vi "PPMS_Measure_v2.vi"(6 "error in (no error)":errorcluster, 7 "Index":i8) -> (0 "error out":errorcluster, 2 "resulting string 1":string="Measure Lockin Channe1, Channel2,  Averages 0 every 0 seconds", 3 "Cancelled?":bool=TRUE)   [LabVIEW 2017]
doc: "Use this template to create a dialog box. This template polls the state of the buttons on the front panel and does not use events. Use the Dialog Using Events template (not available in Base package) to create a dialog box with event handling."
panel:
  in  "Meas Time (s)":dbl=10.0
  in  "Stability timeout (s)":dbl=10.0
  out "MODE":i32(ring) items=["SET&MEAS", "SCAN", ""]
  in  "Measure Rate (s)":dbl=1.0 format="%.3f"
  in  "Averages":u16=10
  in  "Cancel":bool
  in  "OK":bool
  # "Noviembre 2020 V1.2  a-sslcdms"
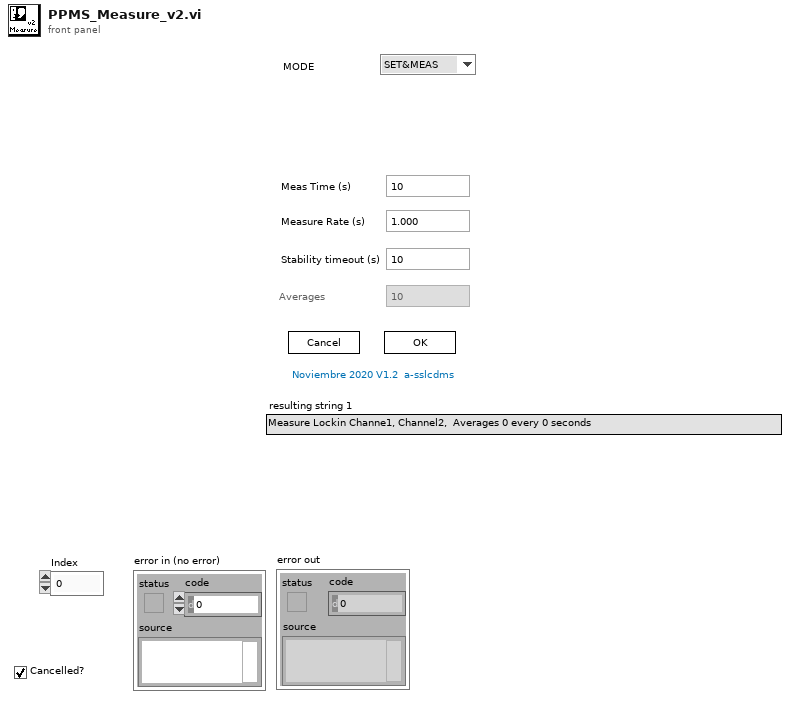
[diagram p1: front panel]
types:
  T1 = enum8{"Enabled", "Disabled", "Disabled and Grayed Out"}
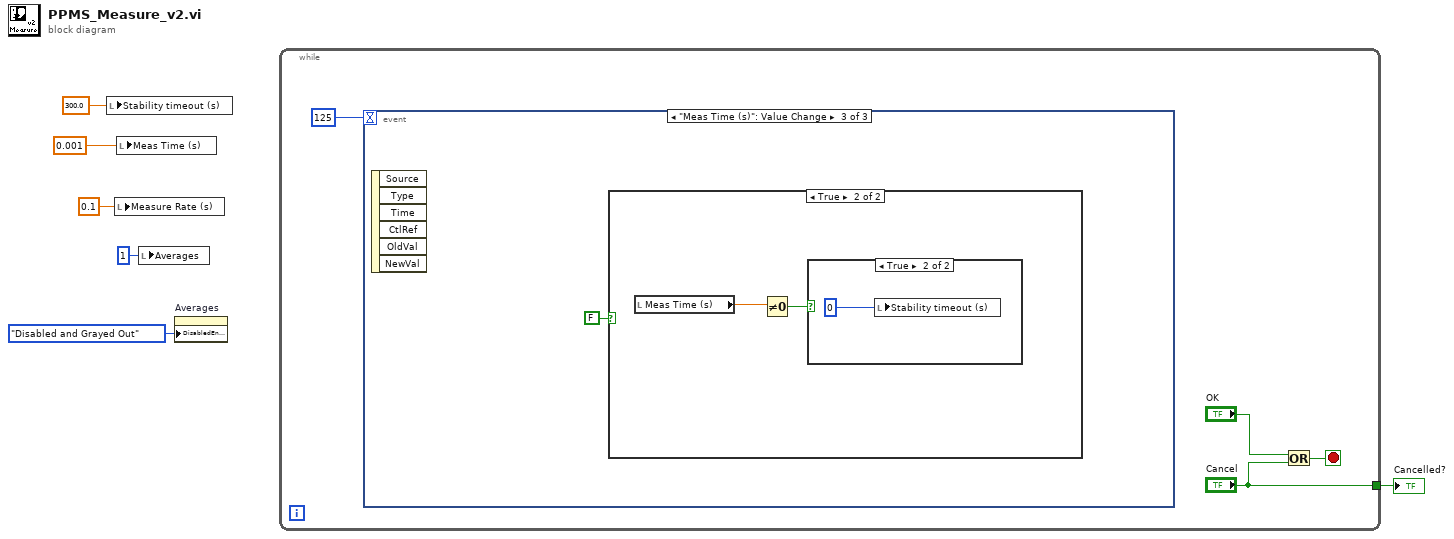
[diagram p0: block diagram]
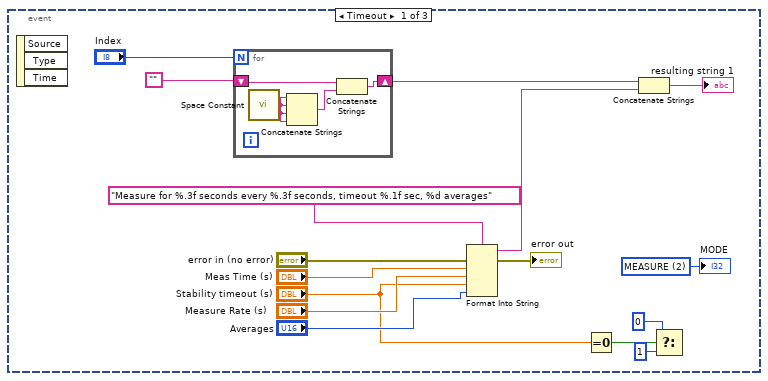
[diagram p2: hidden frame]
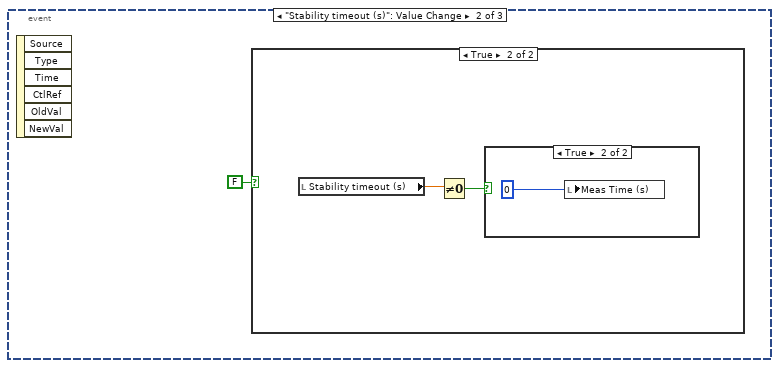
[diagram p3: hidden frame]
diagram:
  n1 = local write "Stability timeout (s)"(300.0 ("#Points (SCAN MODE)")) -> ()
  n2 = local write "Measure Rate (s)"(0.1 ("Measure Rate (sec)")) -> ()
  n3 = local write "Meas Time (s)"(0.001 ("#Points (SCAN MODE)")) -> ()
  n4 = local write "Averages"(u16 1 ("Averages")) -> ()
  n5 = property on="Averages" class="DigNum (strict)"("DisabledEnum"=T1."Disabled and Grayed Out" ("Disabled")) -> ()  [unwired: 2 in, 2 out]
  n6 = while {
    tunnel: ["Cancel"] -> w6
    stop <- w9 stop-if-true
    n7 = event shown="[2] \"Meas Time (s)\": Value Change" {
      selector: _ -> [_ _ _]
      dyn-events: _ -> [_ _ _]
      timeout: 125 -> [_ _ _]
      event Timeout {
        w11 = 2 items=["SET&MEAS", "SCAN", "MEASURE"] ("MODE")
        n8 = event-data() -> ()  [unwired: 1 in, 3 out]
        n9 = for {
          N: "Index" -> [_]
          shift-right: [w29] -> w24
          shift-left: "" -> [w28]
          n10 = call <vilib>:"Space Constant.vi"() -> ("String"=w27:string)
          n11 = Concatenate Strings(w27, w27, w27, w27) -> (w30:string)
          n12 = Concatenate Strings(w28, w30) -> (w29:string)
        }
        n13 = Format Into String(format string="Measure for %.3f seconds every %.3f seconds, timeout %.1f sec, %d averages", error in="error in (no error)", "Meas Time (s)", "Measure Rate (s)", "Stability timeout (s)", "Averages") -> (resulting string=w22:string, error out=→"error out":errorcluster)  [unwired: 1 in]
        n14 = Equal To 0?(x="Stability timeout (s)") -> (x = 0?=w16:bool)
        n15 = Concatenate Strings(w24, w22) -> (→"resulting string 1":string)
        n16 = Select(t=0, s=w16, f=1) -> ()  [unwired: 1 out]
        "MODE" <- w11
      }
      event "Stability timeout (s)": Value Change {
        n17 = event-data() -> ()  [unwired: 1 in, 6 out]
        n18 = case shown="True" FALSE {
          frame False {
          }
          frame True {
            n19 = local read "Stability timeout (s)"() -> (w32:dbl)
            n20 = Not Equal To 0?(x=w32) -> (x != 0?=w33:bool)
            n21 = case shown="True" w33 {
              frame False {
              }
              frame True {
                n22 = local write "Meas Time (s)"(u16 0 ("#Points (SCAN MODE)")) -> ()
              }
            }
          }
        }
      }
      event "Meas Time (s)": Value Change {
        n23 = event-data() -> ()  [unwired: 1 in, 6 out]
        n24 = case shown="True" FALSE {
          frame False {
          }
          frame True {
            n25 = local read "Meas Time (s)"() -> (w37:dbl)
            n26 = Not Equal To 0?(x=w37) -> (x != 0?=w36:bool)
            n27 = case shown="True" w36 {
              frame False {
              }
              frame True {
                n28 = local write "Stability timeout (s)"(u16 0 ("#Points (SCAN MODE)")) -> ()
              }
            }
          }
        }
      }
    }
    n29 = Or(x="OK", y="Cancel") -> (x .or. y?=w9:bool)
  }
  "Cancelled?" <- w6
